vi "Rotation_CreateXY.vi"(9 "Y or sine":dbl, 11 "X or  cosine":dbl) -> (3 "ROTATION":T1)   [LabVIEW 2019, in "Trajectory_Library.lvlib"]
doc: "Constructs a Rotation2d with the given x and y (cosine and sine) components. X and Y don't have to be normalized.\n\nParameters:\n\n - X -The x component or cosine of the rotation.\n - Y - The y component or sine of the rotation.\n\nReturns:\n Rotation data structure"
uses:
  Trajectory_Library.lvlib
  ROTATION2D.ctl
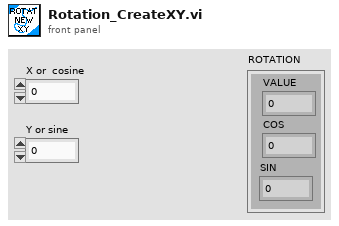
[diagram p1: front panel]
types:
  T1 = typedef "Trajectory_Library.lvlib/ROTATION2D.ctl" = cluster{"VALUE":dbl, "COS":dbl, "SIN":dbl}
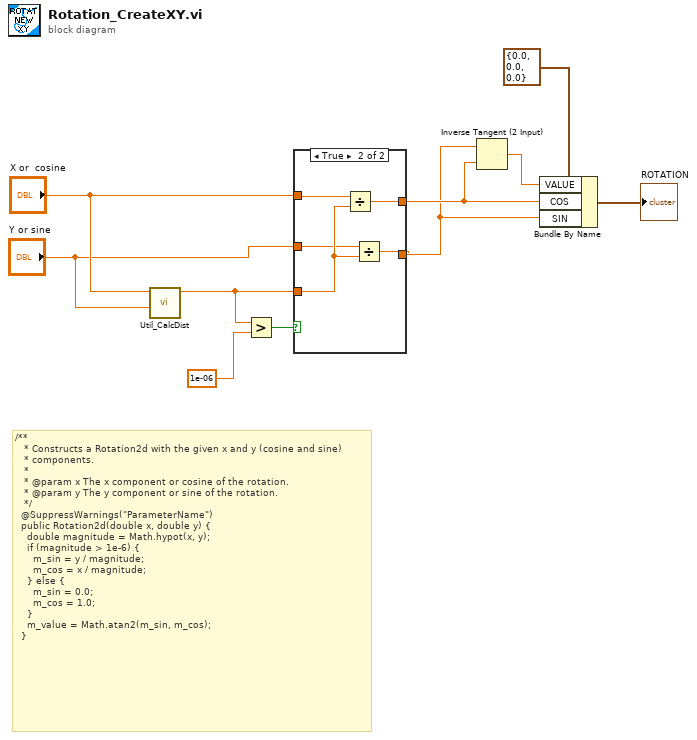
[diagram p0: block diagram]
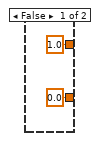
[diagram p2: hidden frame]
diagram:
  # "/**\n   * Constructs a Rotation2d with the given x and y (cosine and sine)\n   * components.\n   *\n   * @param x The x component or cosine of the rotation.\n   * @param y The y component or sine of the rotation.\n   */\n  @SuppressWarnings(\"ParameterName\")\n  public Rotation2d(double x, double y) {\n    double magnitude = Math.hypot(x, y);\n    if (magnitude > 1e-6) {\n      m_sin = y / magnitude;\n      m_cos = x / magnitude;\n    } else {\n      m_sin = 0.0;\n      m_cos = 1.0;\n    }\n    m_value = Math.atan2(m_sin, m_cos);\n  }"
  n1 = call "Util_CalcDist.vi"("Y"="Y or sine", "X"="X or  cosine") -> ("DIST"=w3:dbl)  [unwired: 9 in]
  n2 = Greater?(x=w3, y=1e-06) -> (0:w7:bool)
  n3 = case shown="True" w7 {
    tunnel: "X or  cosine" -> [_ w17]
    tunnel: w3 -> [_ w16]
    tunnel: [1.0 w15] -> w6
    tunnel: "Y or sine" -> [_ w14]
    tunnel: [0.0 w13] -> w5
    frame False {
    }
    frame True {
      n4 = Divide(x=w17, y=w16) -> (x/y=w15:dbl)
      n5 = Divide(x=w14, y=w16) -> (x/y=w13:dbl)
    }
  }
  n6 = Inverse Tangent (2 Input)(1:w6, 2:w5) -> (0:w4:dbl)
  n7 = Bundle By Name(cluster=T1 {"VALUE"=0.0, "COS"=0.0, "SIN"=0.0} ("ROTATION"), "VALUE"=w4, "COS"=w6, "SIN"=w5) -> (→"ROTATION":T1)
